vi "Init.vi"(8 "error in":errorcluster, 11 "IInstrument in":refnum<class "IInstrument.lvclass">) -> (0 "error out":errorcluster, 3 "IInstrument out":refnum<class "IInstrument.lvclass">)   [LabVIEW 2024, in "IInstrument.lvclass"]
uses:
  IInstrument.lvclass
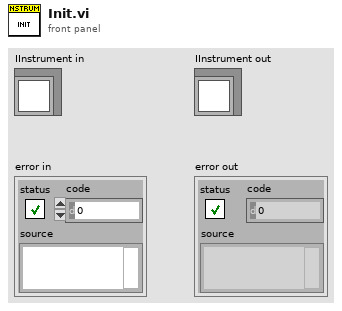
[diagram p1: front panel]
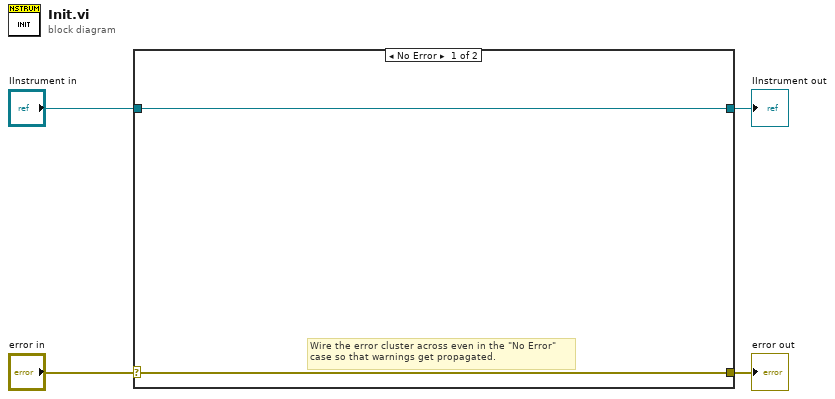
[diagram p0: block diagram]
diagram:
  n1 = case shown="No Error" "error in" {
    selector: "error in" -> [w5 w8]
    tunnel: [w5 w8] -> w3
    tunnel: [w6 w7] -> w1
    tunnel: "IInstrument in" -> [w6 w7]
    frame No Error {
      # "Wire the error cluster across even in the \"No Error\"\ncase so that warnings get propagated."
    }
    frame Error {
    }
  }
  "error out" <- w3
  "IInstrument out" <- w1
